vi "optionen.vi"(9 "shortkatz mit?":bool, 10 "viersualisierung_in":bool, 11 "deutsch?":bool) -> (0 "mit?":bool, 1 "abbgebrochen?":bool, 2 "Viersualisierung?":bool, 3 "Deutsch?":bool)   [LabVIEW 2010]
panel:
  out "data-control refnum out":refnum<vi>
  in  "hilfe":bool
  in  "Einstellungs auswahl":i32(listbox)
  out "ende?":bool=TRUE
  in  "abbrechen":bool
  in  "OK":bool
  out "String":string
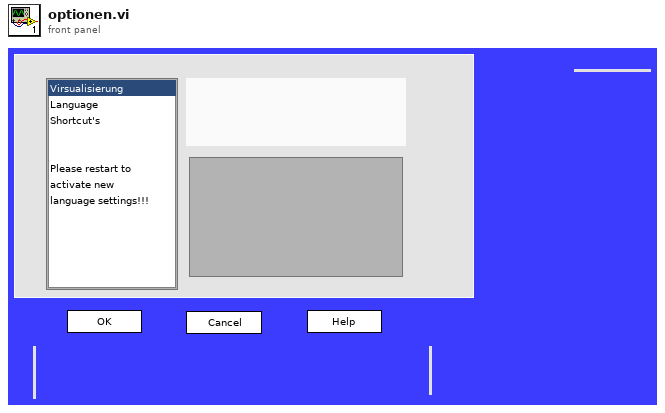
[diagram p1: front panel]
types:
  T1 = typedef "LVPoint32TypeDef.ctl" = cluster{"Horizontal":i32, "Vertical":i32}
  T2 = enum32{"Bad", "Idle", "Run top level", "Running"}
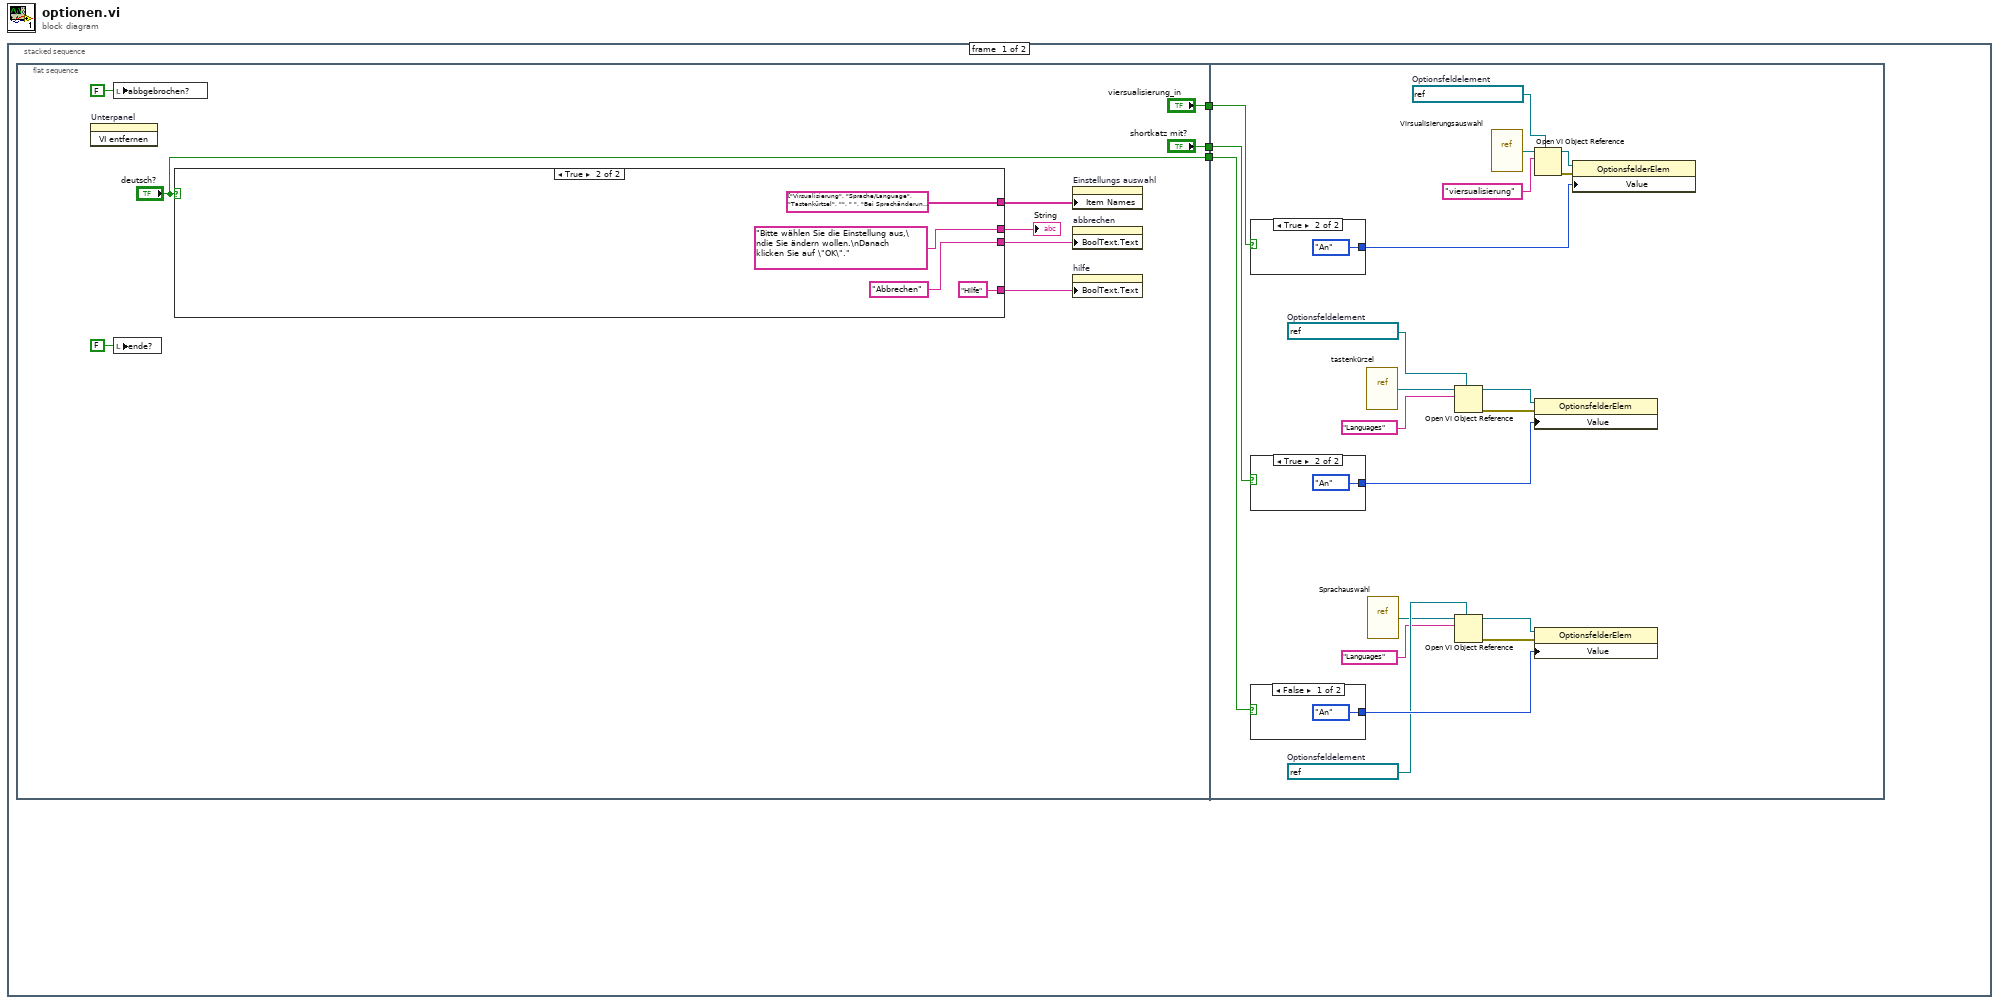
[diagram p0: block diagram]
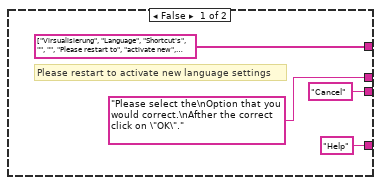
[diagram p2: hidden frame]
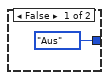
[diagram p3: hidden frame]
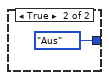
[diagram p4: hidden frame]
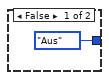
[diagram p5: hidden frame]
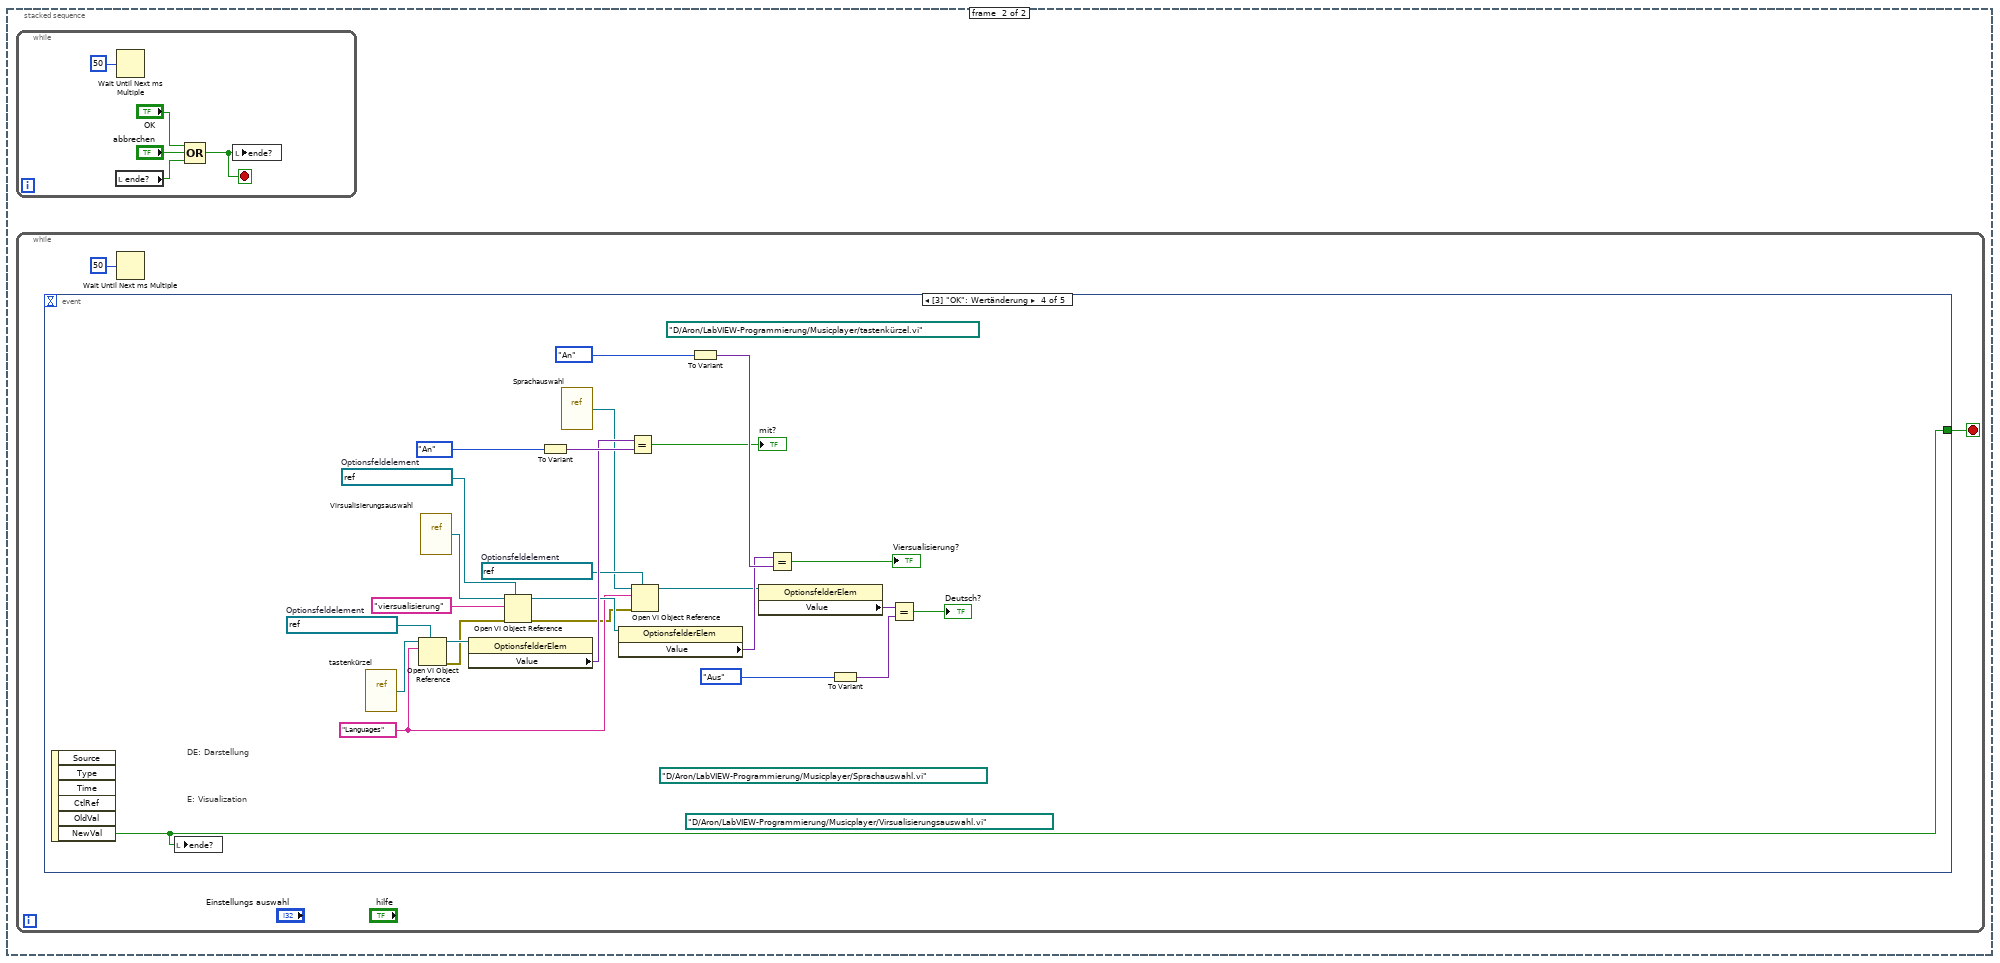
[diagram p6: hidden frame]
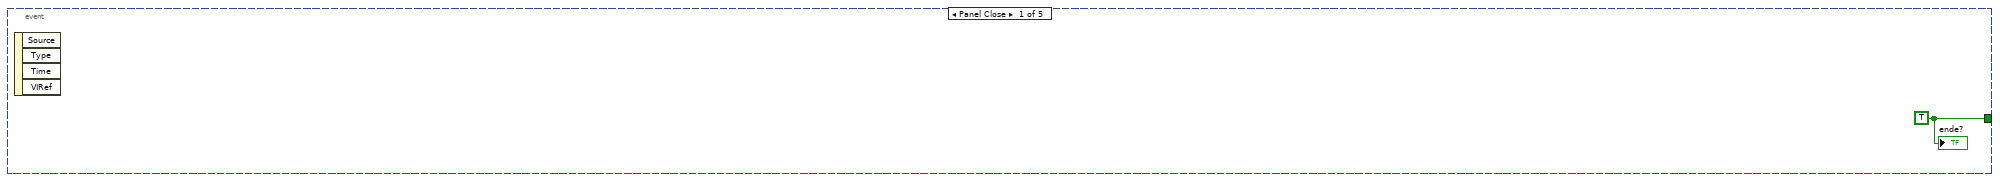
[diagram p7: hidden frame]
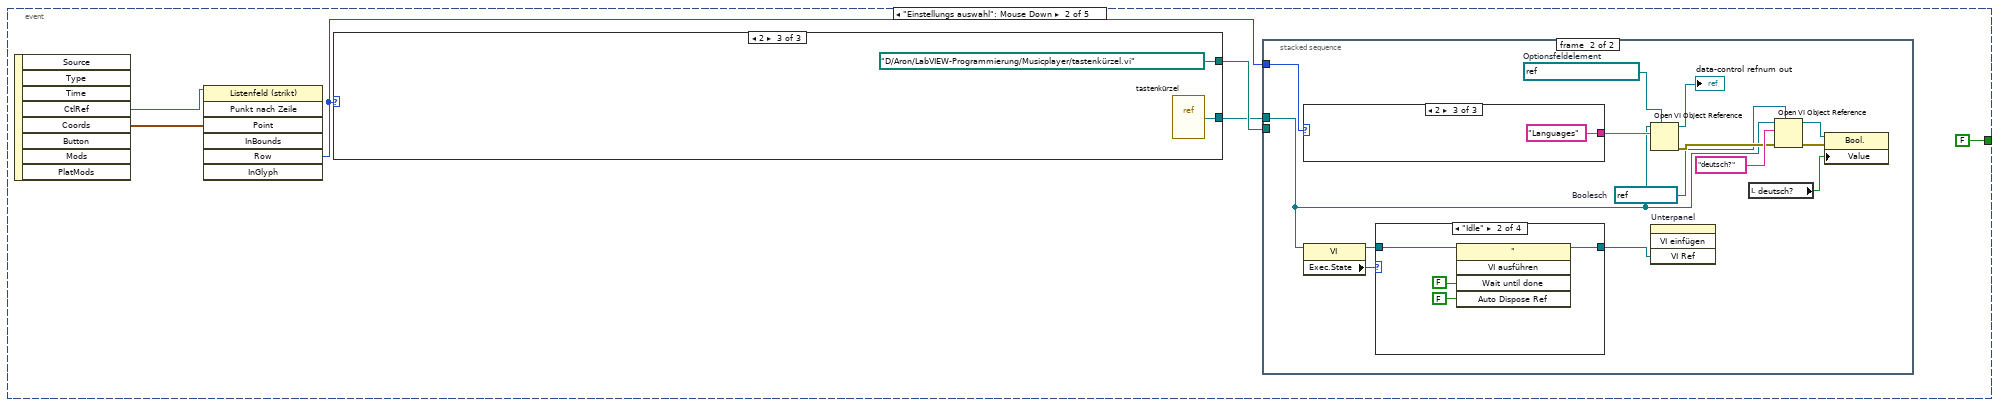
[diagram p8: hidden frame]
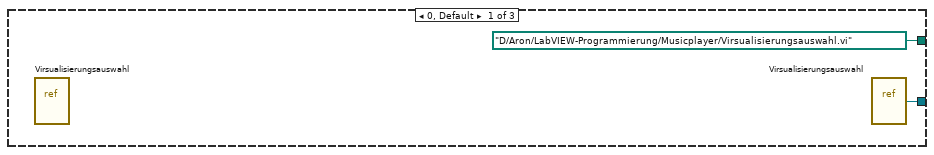
[diagram p9: hidden frame]
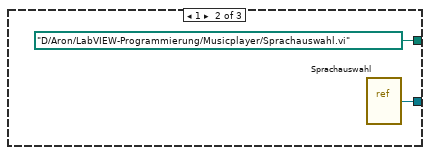
[diagram p10: hidden frame]
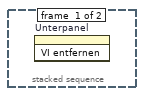
[diagram p11: hidden frame]
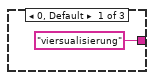
[diagram p15: hidden frame]
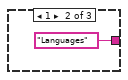
[diagram p16: hidden frame]
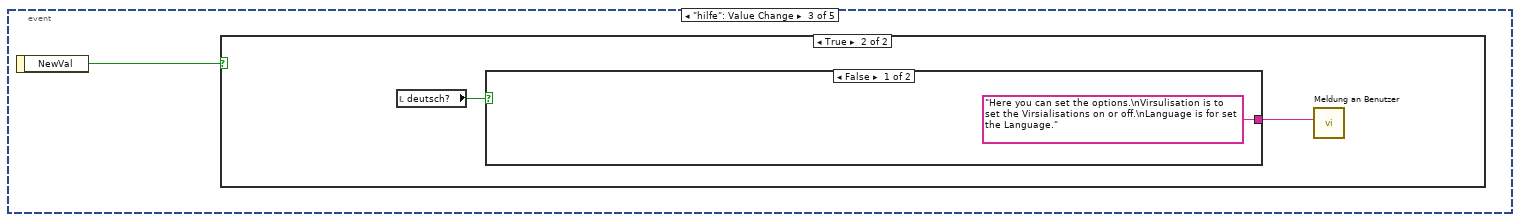
[diagram p17: hidden frame]
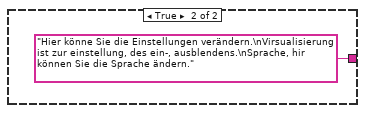
[diagram p19: hidden frame]
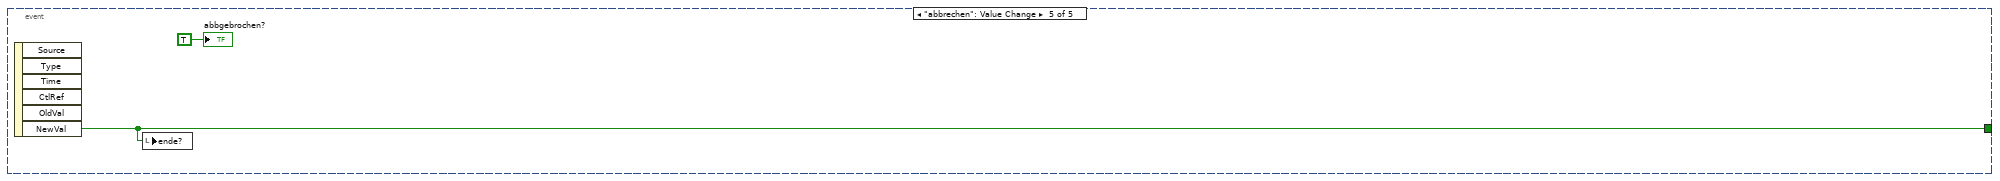
[diagram p20: hidden frame]
diagram:
  n1 = stacked-sequence {
    frame #0 {
      n2 = flat-sequence {
        tunnel: ["deutsch?"] -> w3
        tunnel: ["viersualisierung_in"] -> w2
        tunnel: ["shortkatz mit?"] -> w1
        tunnel: w3 -> [w38]
        tunnel: w2 -> [w40]
        tunnel: w1 -> [w37]
        frame #0 {
          n3 = invoke on="Unterpanel" class="Unterpanel" method="VI entfernen"() -> ()  [unwired: 3 in, 3 out]
          n4 = local write "abbgebrochen?"(FALSE) -> ()
          n5 = local write "ende?"(FALSE) -> ()
          n6 = case shown="True" "deutsch?" {
            tunnel: ["Please select the\nOption that you would correct.\nAfther the correct click on \"OK\"." "Bitte wählen Sie die Einstellung aus,\ndie Sie ändern wollen.\nDanach klicken Sie auf \"OK\"."] -> w12
            tunnel: [string[] ["Virsualisierung", "Language", "Shortcut's", "", "", "Please restart to", "activate new", "language settings!!!"] ("Objektnamen") string[] ["Virsualisierung", "Sprache/Language", "Tastenkürtzel", "", " ", "Bei Sprachänderung", "bitte den Musicplayer", "neu starten, danke!!!"] ("Objektnamen")] -> w11
            tunnel: ["Cancel" "Abbrechen"] -> w6
            tunnel: ["Help" "Hilfe"] -> w5
            frame False {
              # "Please restart to activate new language settings"
            }
            frame True {
            }
          }
          "String" <- w12
          n7 = property on="Einstellungs auswahl" class="Listenfeld (strikt)"("Item Names"=w11) -> ()  [unwired: 2 in, 2 out]
          n8 = property on="abbrechen" class="Bool."("BoolText.Text"=w6) -> ()  [unwired: 2 in, 2 out]
          n9 = property on="hilfe" class="Bool."("BoolText.Text"=w5) -> ()  [unwired: 2 in, 2 out]
        }
        frame #1 {
          w25 = refnum<vi> refnum  # Optionsfeldelement
          w35 = refnum<vi> refnum  # Optionsfeldelement
          w30 = refnum<vi> refnum  # Optionsfeldelement
          n10 = case shown="True" w40 {
            tunnel: [enum32{"An", "Aus"}."Aus" ("Ordner/Datei") enum32{"An", "Aus"}."An" ("Ordner/Datei")] -> w41
            frame False {
            }
            frame True {
            }
          }
          n11 = case shown="True" w37 {
            tunnel: [enum32{"An", "Aus"}."Aus" ("Ordner/Datei") enum32{"An", "Aus"}."An" ("Ordner/Datei")] -> w36
            frame False {
            }
            frame True {
            }
          }
          n12 = case shown="False" w38 {
            tunnel: [enum32{"An", "Aus"}."An" ("Ordner/Datei") enum32{"An", "Aus"}."Aus" ("Ordner/Datei")] -> w39
            frame False {
            }
            frame True {
            }
          }
          n13 = vi-ref "tastenkürzel.vi"() -> (w29:refnum<vi>)
          n14 = vi-ref "Sprachauswahl.vi"() -> (w34:refnum<vi>)
          n15 = Open VI Object Reference(7:w30, 10:"Languages", 11:w29) -> (0:w28:errorcluster, 3:w27:refnum<vi>)  [unwired: 1 in]
          n16 = Open VI Object Reference(7:w35, 10:"Languages", 11:w34) -> (0:w32:errorcluster, 3:w31:refnum<vi>)  [unwired: 1 in]
          n17 = vi-ref "Virsualisierungsauswahl.vi"() -> (w24:refnum<vi>)
          n18 = Open VI Object Reference(7:w25, 10:"viersualisierung", 11:w24) -> (0:w22:errorcluster, 3:w21:refnum<vi>)  [unwired: 1 in]
          n19 = property class="OptionsfelderElem"(reference=w27, error in=w28, "Value"=w36) -> ()  [unwired: 2 out]
          n20 = property class="OptionsfelderElem"(reference=w31, error in=w32, "Value"=w39) -> ()  [unwired: 2 out]
          n21 = property class="OptionsfelderElem"(reference=w21, error in=w22, "Value"=w41) -> ()  [unwired: 2 out]
        }
      }
    }
    frame #1 {
      n22 = while {
        stop <- w120 stop-if-true
        n23 = local read "ende?"() -> (w121:bool)
        n24 = Wait Until Next ms Multiple(millisecond multiple=50) -> ()  [unwired: 1 out]
        n25 = Compound Arithmetic op=OR("OK", "abbrechen", w121) -> (w120:bool)
        n26 = local write "ende?"(w120) -> ()
      }
      n27 = while {
        stop <- w48 stop-if-true
        n28 = event shown="[3] \"OK\": Wertänderung" {
          selector: _ -> [_ _ _ _ _]
          dyn-events: _ -> [_ _ _ _ _]
          timeout: _ -> [_ _ _ _ _]
          tunnel: [w50 FALSE ("NewVal") _ w117 w119] -> w48
          event Panel Close {
            w50 = TRUE
            n29 = event-data() -> ()  [unwired: 5 out]
            "ende?" <- w50
          }
          event "Einstellungs auswahl": Mouse Down {
            n30 = event-data() -> ("CtlRef"=w55:refnum<vi>, "Coords"=w54:T1)  [unwired: 7 out]
            n31 = invoke class="Listenfeld (strikt)" method="Punkt nach Zeile"(reference=w55, "Point"=w54) -> ("Row"=w52:i32)  [unwired: 5 in, 6 out]
            n32 = case shown="2" w52 {
              tunnel: [path "D:/Aron/LabVIEW-Programmierung/Musicplayer/Virsualisierungsauswahl.vi" path "D:/Aron/LabVIEW-Programmierung/Musicplayer/Sprachauswahl.vi" path "D:/Aron/LabVIEW-Programmierung/Musicplayer/tastenkürzel.vi"] -> w53
              tunnel: [w57 w59 w61] -> w51
              frame 0, Default {
                n33 = vi-ref "Virsualisierungsauswahl.vi"() -> ()  [unwired: 1 out]
                n34 = vi-ref "Virsualisierungsauswahl.vi"() -> (w57:refnum<vi>)
              }
              frame 1 {
                n35 = vi-ref "Sprachauswahl.vi"() -> (w59:refnum<vi>)
              }
              frame 2 {
                n36 = vi-ref "tastenkürzel.vi"() -> (w61:refnum<vi>)
              }
            }
            n37 = stacked-sequence {
              tunnel: w53 -> [_ _]
              tunnel: w52 -> [_ w76]
              tunnel: w51 -> [_ w66]
              frame #0 {
                n38 = invoke on="Unterpanel" class="SubPanel" method="VI entfernen"() -> ()  [unwired: 3 in, 3 out]
              }
              frame #1 {
                w64 = refnum<vi> refnum  # Optionsfeldelement
                w65 = refnum<vi> refnum  # Boolesch
                n39 = case shown="2" w76 {
                  tunnel: ["viersualisierung" "Languages" "Languages"] -> w68
                  frame 0, Default {
                  }
                  frame 1 {
                  }
                  frame 2 {
                  }
                }
                n40 = property class="VI"(reference=w66) -> (reference out=w72:refnum<vi>, "Exec.State"=w74:T2)  [unwired: 1 in, 1 out]
                n41 = case shown="\"Idle\"" w74 {
                  tunnel: [w77 w79 w82 w83] -> w73
                  tunnel: w72 -> [w77 w78 w82 w83]
                  frame "Bad", Default {
                  }
                  frame "Idle" {
                    n42 = invoke class="\"" method="VI ausführen"(reference=w78, "Wait until done"=FALSE ("Warten bis beendet"), "Auto Dispose Ref"=FALSE ("Referenz automatisch schließen")) -> (reference out=w79:refnum<vi>)  [unwired: 2 in, 4 out]
                  }
                  frame "Run top level" {
                  }
                  frame "Running" {
                  }
                }
                n43 = Open VI Object Reference(7:w64, 10:w68, 11:w66) -> (0:w67:errorcluster, 3:→"data-control refnum out":refnum<vi>)  [unwired: 1 in]
                n44 = invoke on="Unterpanel" class="SubPanel" method="VI einfügen"("VI Ref"=w73) -> ()  [unwired: 3 in, 4 out]
                n45 = local read "deutsch?"() -> (w75:bool)
                n46 = Open VI Object Reference(7:w65, 8:w67, 10:"deutsch?" ("control name"), 11:w66) -> (0:w70:errorcluster, 3:w69:refnum<vi>)
                n47 = property class="Bool."(reference=w69, error in=w70, "Value"=w75) -> ()  [unwired: 2 out]
              }
            }
          }
          event "hilfe": Value Change {
            n48 = event-data() -> ("NewVal"=w87:bool)  [unwired: 1 out]
            n49 = case shown="True" w87 {
              frame False {
              }
              frame True {
                n50 = local read "deutsch?"() -> (w89:bool)
                n51 = case shown="False" w89 {
                  tunnel: ["Here you can set the options.\nVirsulisation is to set the Virsialisations on or off.\nLanguage is for set the Language." "Hier könne Sie die Einstellungen verändern.\nVirsualisierung ist zur einstellung, des ein-, ausblendens.\nSprache, hir können Sie die Sprache ändern."] -> w88
                  frame False {
                  }
                  frame True {
                  }
                }
                n52 = call "Meldung an Benutzer"("Message"=w88) -> ()  [unwired: 2 in, 9 out]
              }
            }
          }
          event "OK": Value Change {
            w96 = refnum<vi> refnum  # Optionsfeldelement
            w101 = refnum<vi> refnum  # Optionsfeldelement
            w104 = refnum<vi> refnum  # Optionsfeldelement
            (unwired) path "D:/Aron/LabVIEW-Programmierung/Musicplayer/tastenkürzel.vi"
            (unwired) path "D:/Aron/LabVIEW-Programmierung/Musicplayer/Sprachauswahl.vi" ("path")
            (unwired) path "D:/Aron/LabVIEW-Programmierung/Musicplayer/Virsualisierungsauswahl.vi" ("path")
            w95 = "Languages"
            # "E: Visualization"
            # "DE: Darstellung"
            n53 = event-data() -> ("NewVal"=w117:bool)  [unwired: 6 out]
            n54 = local write "ende?"(w117) -> ()
            n55 = vi-ref "tastenkürzel.vi"() -> (w103:refnum<vi>)
            n56 = Open VI Object Reference(7:w104, 10:w95, 11:w103) -> (0:w98:errorcluster, 3:w102:refnum<vi>)  [unwired: 1 in]
            n57 = vi-ref "Virsualisierungsauswahl.vi"() -> (w100:refnum<vi>)
            n58 = property class="OptionsfelderElem"(reference=w102) -> ("Value"=w106:variant)  [unwired: 1 in, 2 out]
            n59 = Open VI Object Reference(7:w101, 8:w98, 10:"viersualisierung", 11:w100) -> (0:w93:errorcluster, 3:w97:refnum<vi>)
            n60 = To Variant(anything=enum32{"An", "Aus"}."An" ("Ordner/Datei")) -> (Variant=w108:variant)
            n61 = vi-ref "Sprachauswahl.vi"() -> (w94:refnum<vi>)
            n62 = property class="OptionsfelderElem"(reference=w97) -> ("Value"=w115:variant)  [unwired: 1 in, 2 out]
            n63 = Equal?(x=w106, y=w108) -> (x = y?=→"mit?":bool)
            n64 = Open VI Object Reference(7:w96, 8:w93, 10:w95, 11:w94) -> (3:w92:refnum<vi>)  [unwired: 1 out]
            n65 = To Variant(anything=enum32{"An", "Aus"}."An" ("Ordner/Datei")) -> (Variant=w116:variant)
            n66 = property class="OptionsfelderElem"(reference=w92) -> ("Value"=w112:variant)  [unwired: 1 in, 2 out]
            n67 = Equal?(x=w115, y=w116) -> (x = y?=→"Viersualisierung?":bool)
            n68 = To Variant(anything=enum32{"An", "Aus"}."Aus" ("Ordner/Datei")) -> (Variant=w113:variant)
            n69 = Equal?(x=w112, y=w113) -> (x = y?=→"Deutsch?":bool)
          }
          event "abbrechen": Value Change {
            n70 = event-data() -> ("NewVal"=w119:bool)  [unwired: 6 out]
            n71 = local write "ende?"(w119) -> ()
            "abbgebrochen?" <- TRUE ("abbgebrochen?")
          }
        }
        n72 = Wait Until Next ms Multiple(millisecond multiple=50) -> ()  [unwired: 1 out]
      }
    }
  }
